vi "publish status.vi"(8 "error in (no error)":errorcluster, 11 "S4GEI in":refnum<class "S4GEI.lvclass">) -> (0 "error out":errorcluster, 3 "S4GEI out":refnum<class "S4GEI.lvclass">)   [LabVIEW 2018, in "S4GEI.lvclass"]
uses:
  S4GEI.lvclass
  S4GEI.lvclass/S4GEI.ctl
  State Machine/State Machine.lvclass/State Machine.ctl
  State Machine/State Machine.lvclass
  RxTx/RxTx.lvclass
  S4ICS/S4ICS.lvclass
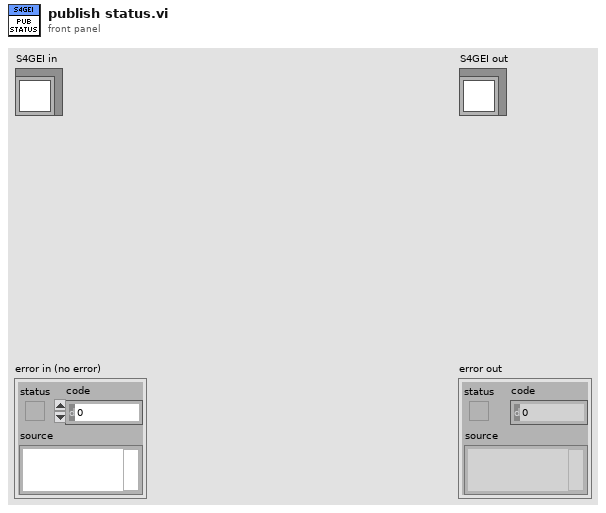
[diagram p1: front panel]
types:
  T1 = cluster{"OBJECT":string, "OBSERVER":string, "CTRLINTE":string, "PROJID":string, "SYNCMODE":string, "INSTMODE":string, "FILTER":string, "OBSTYPE":string, "GUIVRSN":string, "COMMENT":string, "broker":string, "timestamp":string, "CHANNEL 1":bool, "CHANNEL 2":bool, "CHANNEL 3":bool, "CHANNEL 4":bool, "TCSMODE":bool}
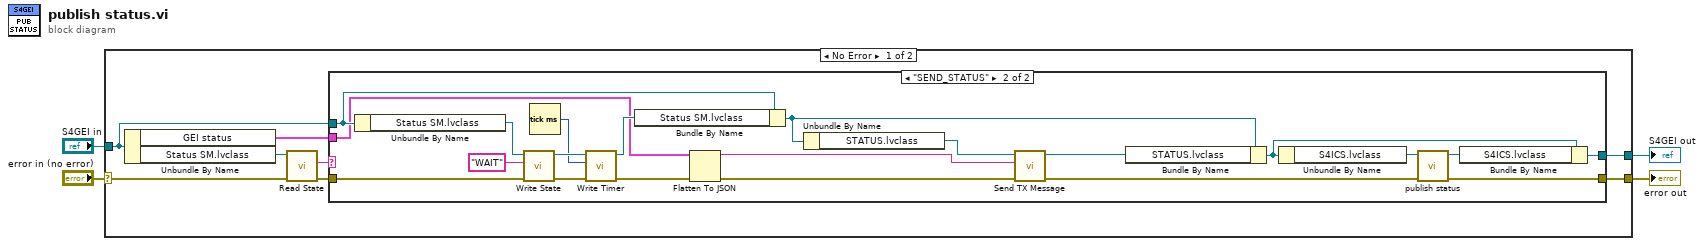
[diagram p0: block diagram]
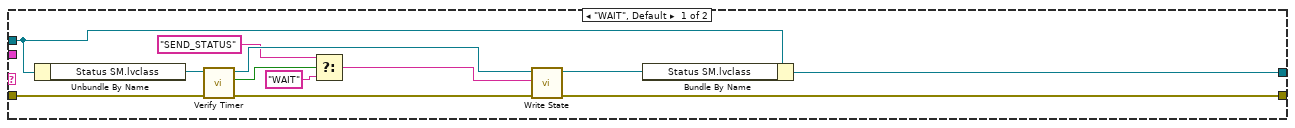
[diagram p2: hidden frame]
diagram:
  n1 = case shown="No Error" "error in (no error)" {
    selector: "error in (no error)" -> [w11 w47]
    tunnel: [w8 w47] -> w3
    tunnel: [w6 w46] -> w1
    tunnel: "S4GEI in" -> [w7 w46]
    frame No Error {
      n2 = Unbundle By Name(w7) -> ("GEI status"=w5:T1, "Status SM.lvclass"=w12:refnum<class "State Machine.lvclass">)
      n3 = call-dynamic "Read State.vi"("error in (no error)"=w11, "State Machine in"=w12) -> ("error out"=w10:errorcluster, "State"=w9:string)  [unwired: 7 in, 1 out]
      n4 = case shown="\"SEND_STATUS\"" w9 {
        tunnel: w10 -> [w17 w40]
        tunnel: [w16 w27] -> w8
        tunnel: w7 -> [w14 w38]
        tunnel: [w13 w28] -> w6
        tunnel: w5 -> [_ w32]
        frame "WAIT", Default {
          n5 = Unbundle By Name(w14) -> ("Status SM.lvclass"=w15:refnum<class "State Machine.lvclass">)
          n6 = call "Verify Timer.vi"("error in (no error)"=w17, "State Machine in"=w15) -> ("error out"=w24:errorcluster, "time out"=w18:bool, "State Machine out"=w23:refnum<class "State Machine.lvclass">)  [unwired: 7 in]
          n7 = Select(t="SEND_STATUS", s=w18, f="WAIT") -> (s? t:f=w21:string)
          n8 = call-dynamic "Write State.vi"("error in (no error)"=w24, "State"=w21, "State Machine in"=w23) -> ("error out"=w16:errorcluster, "State Machine out"=w22:refnum<class "State Machine.lvclass">)  [unwired: 7 in]
          n9 = Bundle By Name(cluster=w14, "Status SM.lvclass"=w22) -> (w13:refnum<class "S4GEI.lvclass">)
        }
        frame "SEND_STATUS" {
          n10 = Unbundle By Name(w38) -> ("Status SM.lvclass"=w41:refnum<class "State Machine.lvclass">)
          n11 = call-dynamic "Write State.vi"("error in (no error)"=w40, "State"="WAIT", "State Machine in"=w41) -> ("error out"=w44:errorcluster, "State Machine out"=w45:refnum<class "State Machine.lvclass">)  [unwired: 7 in]
          n12 = Tick Count (ms)() -> (millisecond timer value=w43:u32)
          n13 = call "Write Timer.vi"("error in (no error)"=w44, "Timer"=w43, "State Machine in"=w45) -> ("error out"=w33:errorcluster, "State Machine out"=w39:refnum<class "State Machine.lvclass">)  [unwired: 7 in]
          n14 = Bundle By Name(cluster=w38, "Status SM.lvclass"=w39) -> (w35:refnum<class "S4GEI.lvclass">)
          n15 = Flatten To JSON(anything=w32, error in (no error)=w33) -> (JSON string=w31:string, 11:w34:errorcluster)  [unwired: 1 in]
          n16 = Unbundle By Name(w35) -> ("STATUS.lvclass"=w37:refnum<class "RxTx.lvclass">)
          n17 = call "Send TX Message.vi"("error in (no error)"=w34, "element"=w31, "RxTx in"=w37) -> ("error out"=w26:errorcluster, "RxTx out"=w36:refnum<class "RxTx.lvclass">)  [unwired: 7 in]
          n18 = Bundle By Name(cluster=w35, "STATUS.lvclass"=w36) -> (w29:refnum<class "S4GEI.lvclass">)
          n19 = Unbundle By Name(w29) -> ("S4ICS.lvclass"=w30:refnum<class "S4ICS.lvclass">)
          n20 = call "publish status.vi"("error in (no error)"=w26, "S4ICS in"=w30) -> ("error out"=w27:errorcluster, "S4ICS out"=w25:refnum<class "S4ICS.lvclass">)  [unwired: 8 in]
          n21 = Bundle By Name(cluster=w29, "S4ICS.lvclass"=w25) -> (w28:refnum<class "S4GEI.lvclass">)
        }
      }
    }
    frame Error {
    }
  }
  "error out" <- w3
  "S4GEI out" <- w1
